vi "Processor Link Status.vi"(0 "fpga reference in":T1, 11 "error in":errorcluster) -> (4 "fpga reference out":T1, 6 "link status":T2(array[cluster]) {"Lane Up" format="%.0b"}, 8 "healthy link":bool[](array[boolean]), 15 "error out":errorcluster)   [LabVIEW 2019]
uses:
  TypeDefs/Blank FPGA Reference.ctl
  TypeDefs/Processor FPGA Reference.ctl
  <vilib>/Utility/error.llb/Error Cluster From Error Code.vi
  <vilib>/rvi/errors/niLvFpgaAdjustHostInterfaceError.vi
  <vilib>/rvi/interface/nirviReadWriteControl/nirviReadWriteControl.xnode
  NiFpgaLv.dll
  <vilib>/rvi/interface/Simulation/niFpgaSimulationCallBeginRW.vi
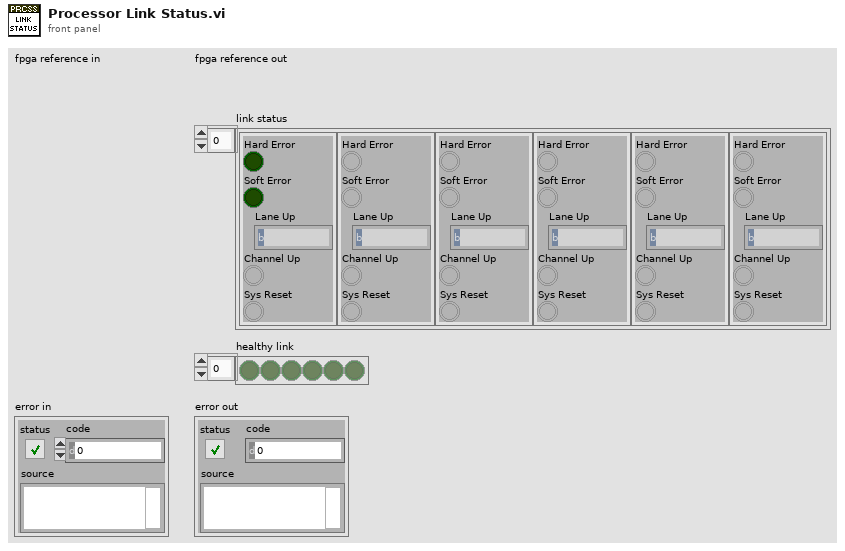
[diagram p1: front panel]
types:
  T1 = typedef "Blank FPGA Reference.ctl" = refnum<k20>
  T2 = cluster{"Hard Error":bool, "Soft Error":bool, "Lane Up":fxp<+,4,4>, "Channel Up":bool, "Sys Reset":bool}[]
  T3 = typedef "Processor FPGA Reference.ctl" = refnum<k20>
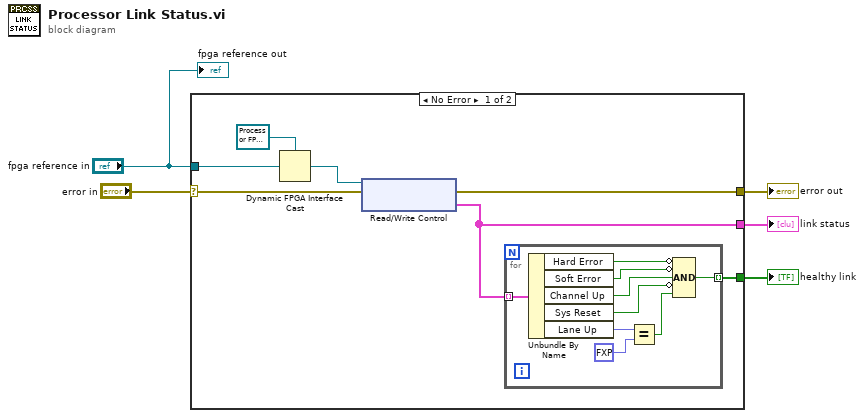
[diagram p0: block diagram]
diagram:
  n1 = case shown="No Error" "error in" {
    selector: "error in" -> [w8 w22]
    tunnel: "fpga reference in" -> [w10 _]
    tunnel: [w9 w22] -> w4
    tunnel: [w6 _] -> w3
    tunnel: [w7 _] -> w1
    frame No Error {
      n2 = Dynamic FPGA Interface Cast(Session In=T3 refnum ("fpga reference"), Type=w10) -> (Session Out=w11:T3)
      n3 = xnode "Read/Write Control"("FPGA VI Reference In"=w11, "error in"=w8) -> ("error out"=w9:errorcluster, "channel status"=w6:T2)  [unwired: 1 out]
      n4 = for {
        tunnel: w6 -> [w21] mode=indexing
        tunnel: [w13] -> w7 mode=indexing
        n5 = Unbundle By Name(w21) -> ("Hard Error"=w18:bool, "Soft Error"=w17:bool, "Channel Up"=w16:bool, "Sys Reset"=w15:bool, "Lane Up"=w20:fxp<+,4,4>)
        n6 = Equal?(x=w20, y=fxp<+,4,4> 15.0) -> (x = y?=w14:bool)
        n7 = Compound Arithmetic op=AND(invert w18, invert w17, w16, invert w15, w14) -> (w13:bool)
      }
    }
    frame Error {
    }
  }
  "error out" <- w4
  "link status" <- w3
  "healthy link" <- w1
  "fpga reference out" <- "fpga reference in"
